vi "Draw Steering Wheel Forward Velocity.vi"(6 "wheel state":T1, 7 "picture info":T3={"picture size"={"Width"=500, "Height"=500}, "pixels per unit"=10.0}, 8 "error in (no error)":errorcluster, 9 "draw wheel options":T2={"global wheel position"={"x"=0.0, "y"=0.0}, "wheel frame angle (rad)"=0.0, "color (black)"=0, "draw wheel state"=FALSE, "draw forward velocity"=FALSE, "velocity scale"=16711680.0, "velocity color (red)"=16711680}, 10 "picture in":picture, 11 "wheel in":refnum<class "NI_Robotics_Wheel.lvclass">) -> (0 "error out":errorcluster, 2 "picture out":picture, 3 "wheel out":refnum<class "NI_Robotics_Wheel.lvclass">)   [LabVIEW 2017, in "NI_Robotics_Steering Picture.lvlib"]
uses:
  <vilib>/robotics/Utilities/Visualization/Steering Visualization/Steering Picture/NI_Robotics_Steering Picture.lvlib
  <vilib>/robotics/Utilities/Visualization/Steering Visualization/Steering Picture/Picture Info.ctl
  <vilib>/Utility/miscctls.llb/LVBoundsTypeDef.ctl
  <vilib>/robotics/Utilities/Visualization/Steering Visualization/Steering Picture/Draw Wheel Options.ctl
  <vilib>/robotics/Steering/Wheel/Wheel State.ctl
  <vilib>/robotics/Steering/Wheel/NI_Robotics_Wheel.lvclass
  <vilib>/Analysis/coordinate.llb/Angle Rotation (scalar).vi
  <vilib>/Analysis/coordinate.llb/2D Cartesian Coordinate Rotation.vi
  <vilib>/Analysis/coordinate.llb/2D Cartesian Coordinate Rotation (Array).vi
  <vilib>/robotics/Utilities/Visualization/Steering Visualization/Steering Picture/Global Position to Pixel.vi
  <vilib>/Analysis/coordinate.llb/Wrap Angle (scalar).vi
  <vilib>/picture/picture.llb/Draw Line.vi
  <vilib>/picture/picture.llb/Move Pen.vi
  <vilib>/Analysis/NI_AAL_Angle.lvlib
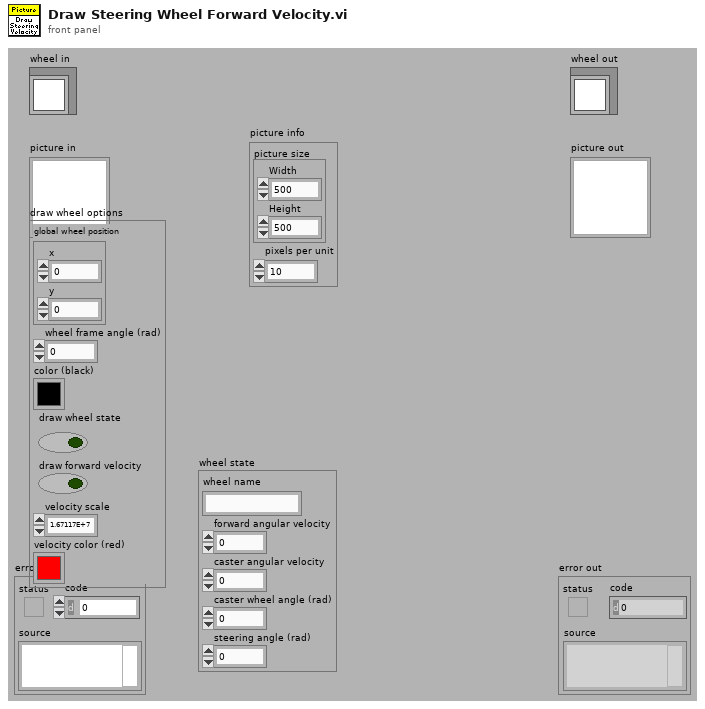
[diagram p1: front panel]
types:
  T1 = typedef "NI_Robotics_Wheel.lvclass/Wheel State.ctl" = cluster{"wheel name":string, "forward angular velocity":dbl, "caster angular velocity":dbl, "caster wheel angle (rad)":dbl, "steering angle (rad)":dbl}
  T2 = typedef "NI_Robotics_Steering Picture.lvlib/Draw Wheel Options.ctl" = cluster{"global wheel position":cluster{"x":dbl, "y":dbl}, "wheel frame angle (rad)":dbl, "color (black)":u32, "draw wheel state":bool, "draw forward velocity":bool, "velocity scale":dbl, "velocity color (red)":u32}
  T3 = typedef "NI_Robotics_Steering Picture.lvlib/Picture Info.ctl" = cluster{"picture size":T4, "pixels per unit":dbl}
  T4 = typedef "LVBoundsTypeDef.ctl" = cluster{"Width":u32, "Height":u32}
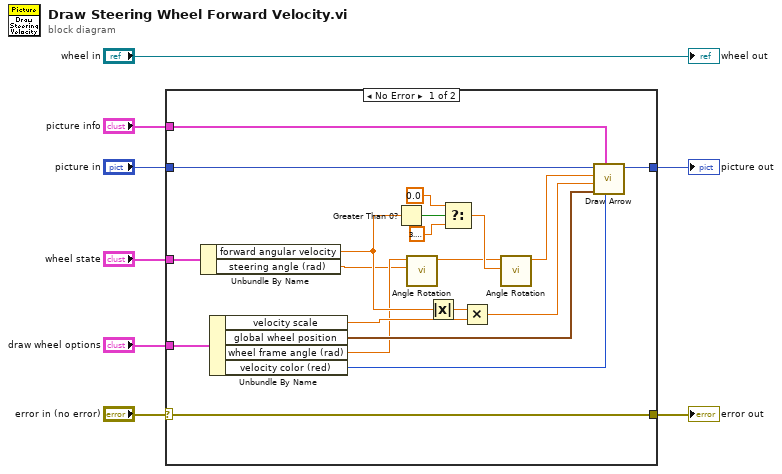
[diagram p0: block diagram]
diagram:
  n1 = case shown="No Error" "error in (no error)" {
    selector: "error in (no error)" -> [w28 w30]
    tunnel: [w28 w30] -> w5
    tunnel: "picture in" -> [w27 w29]
    tunnel: [w26 w29] -> w6
    tunnel: "picture info" -> [w25 _]
    tunnel: "draw wheel options" -> [w24 _]
    tunnel: "wheel state" -> [w22 _]
    frame No Error {
      n2 = Unbundle By Name(w22) -> ("forward angular velocity"=w17:dbl, "steering angle (rad)"=w9:dbl)
      n3 = Unbundle By Name(w24) -> ("velocity scale"=w14:dbl, "global wheel position"=w23:cluster{"x":dbl, "y":dbl}, "wheel frame angle (rad)"=w11:dbl, "velocity color (red)"=w21:u32)
      n4 = Greater Than 0?(x=w17) -> (x > 0?=w18:bool)
      n5 = call-poly <vilib>:"Angle Rotation.vi"("counterclockwise rotation"=w9, "angle"=w11) -> ("rotated angle"=w10:dbl)  [unwired: 8 in, 1 out]
      n6 = Absolute Value(x=w17) -> (abs(x)=w16:dbl)
      n7 = Select(t=0.0, s=w18, f=3.141592653589793) -> (s? t:f=w12:dbl)
      n8 = Multiply(x=w16, y=w14) -> (x*y=w15:dbl)
      n9 = call-poly <vilib>:"Angle Rotation.vi"("counterclockwise rotation"=w12, "angle"=w10) -> ("rotated angle"=w13:dbl)  [unwired: 8 in, 1 out]
      n10 = call <vilib>:"Draw Arrow.vi"("color"=w21, "picture info"=w25, "global base position"=w23, "length"=w15, "wheel frame angle (rad)"=w13, "picture in"=w27) -> ("picture out"=w26:picture)  [unwired: 5 in]
    }
    frame Error {
    }
  }
  "error out" <- w5
  "picture out" <- w6
  "wheel out" <- "wheel in"
